vi "Write Housing Colors.vi"(5 "Housing Colors":T1, 9 "NumericWithScale in":refnum<class "NumericWithScale.lvclass">) -> (3 "NumericWithScale out":refnum<class "NumericWithScale.lvclass">)   [LabVIEW 2014, in "NumericWithScale.lvclass"]
uses:
  NumericWithScale.lvclass
  <vilib>/Utility/miscctls.llb/LVForegroundBackgroundColorsTypeDef.ctl
  NumericWithScale.lvclass/NumericWithScale.ctl
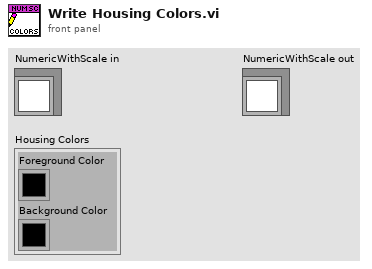
[diagram p1: front panel]
types:
  T1 = typedef "LVForegroundBackgroundColorsTypeDef.ctl" = cluster{"Foreground Color":u32, "Background Color":u32}
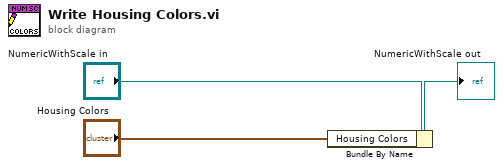
[diagram p0: block diagram]
diagram:
  n1 = Bundle By Name(cluster="NumericWithScale in", "Housing Colors"="Housing Colors") -> (→"NumericWithScale out":refnum<class "NumericWithScale.lvclass">)
